vi "Latihan 2 (Suhu).vi"() -> ()   [LabVIEW 2021]
panel:
  out "Reamur":dbl(slide) scale=0.0..80.0
  out "Kelvin":dbl(slide) scale=273.15..373.15
  in  "Farenheit":dbl(slide) scale=32.0..212.0
  out "Celcius":dbl(slide) scale=0.0..100.0
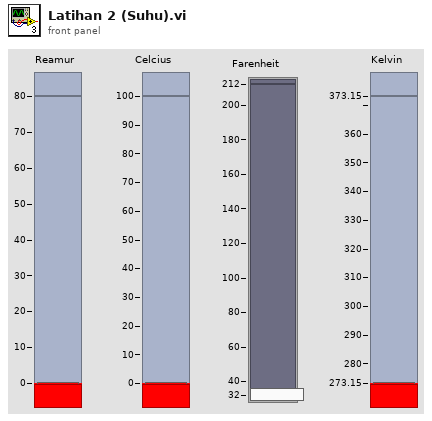
[diagram p1: front panel]
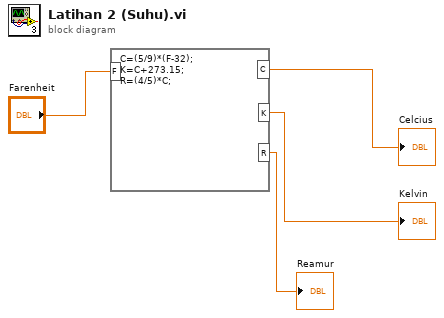
[diagram p0: block diagram]
diagram:
  n1 = formula code="C=(5/9)*(F-32);\nK=C+273.15;\nR=(4/5)*C;"("F"="Farenheit") -> ("C"=→"Celcius":dbl, "K"=→"Kelvin":dbl, "R"=→"Reamur":dbl)
